vi "Sector Analysis Module.vi"(11 "Canceled?":bool) -> (2 "State":T1, 3 "Data":bool, 4 "Left Sector Edge":u8, 5 "Right Sector Edge":u8)   [LabVIEW 2013]
uses:
  Sector Analysis Module Enum.ctl
  <vilib>/rvi/FIFO/Fifo_Resource/nirvififoEmulationReadFpgaImpl.vi
  <vilib>/rvi/DataTransferAndStorage/Container/Common/niFpgaContainerGetUniqueNameForEmu.vi
  Globals/Sector Parameter Global.vi
  <vilib>/rvi/Emulation/niFpgaSctlEmulationGetInTimedLoop.vi
  <vilib>/rvi/Emulation/niFpgaProcessEmulError.vi
  Globals/Accumulated Sector Intensity.vi
  <vilib>/rvi/FIFO/Fifo_Resource/nirvififoEmulationClearFpgaImpl.vi
  <vilib>/rvi/DataTransferAndStorage/Container/XNode/niFpgaContainer.xnode
  <vilib>/rvi/FIFO/Fifo_Resource/nirvififoEmulationRead.vi
  <vilib>/rvi/FIFO/Fifo_Resource/nirvififoEmulationClear.vi
panel:
  out "2nd Analysis Left Sector":u8
  out "2nd Analysis Right Sector":u8
  out "Preanalysis Right Sector Edge":u8
  out "Preanalysis Left Sector Edge":u8
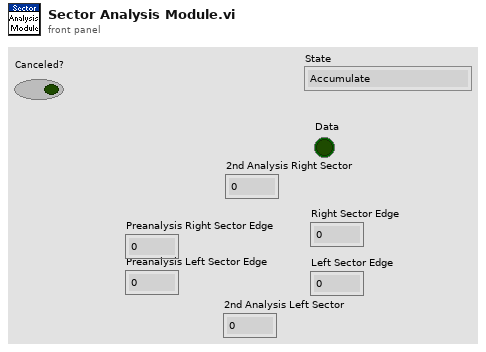
[diagram p1: front panel]
types:
  T1 = typedef "Sector Analysis Module Enum.ctl" = enum16{"Accumulate", "Analysis", "Reset"}
  T2 = typedef "Sector Parameter Cluster.ctl" = cluster{"Start Angle":fxp<+/-,17,2>, "End Angle":fxp<+/-,17,2>, "Inner Radius":u16, "Outter Radius":u16, "Hinge X":u16, "Hinge Y":u16, "NumWingSectors":u8}
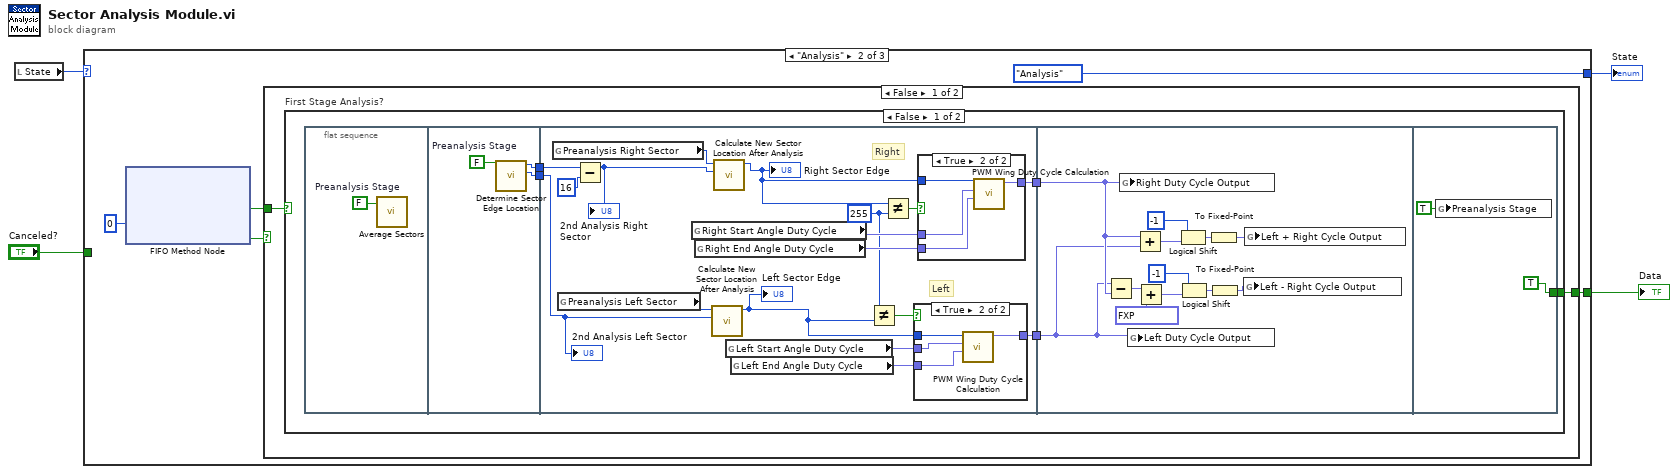
[diagram p0: block diagram]
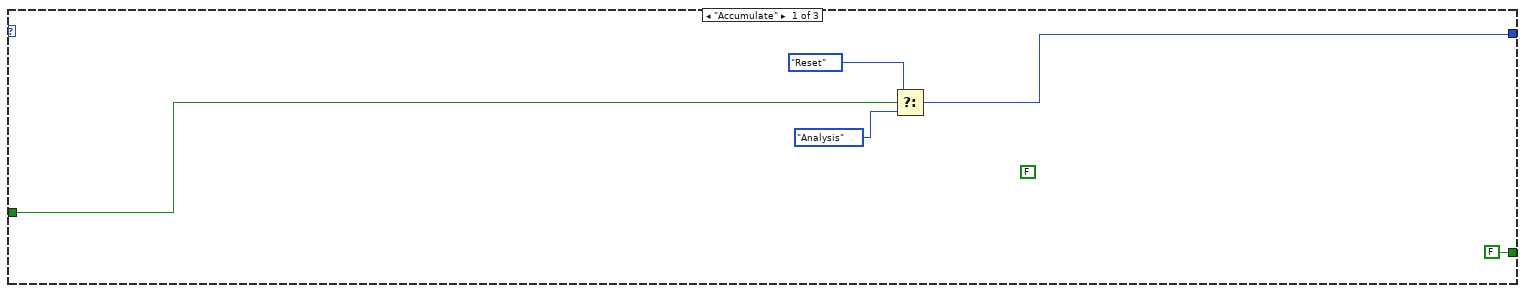
[diagram p2: hidden frame]
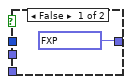
[diagram p3: hidden frame]
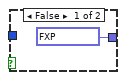
[diagram p4: hidden frame]
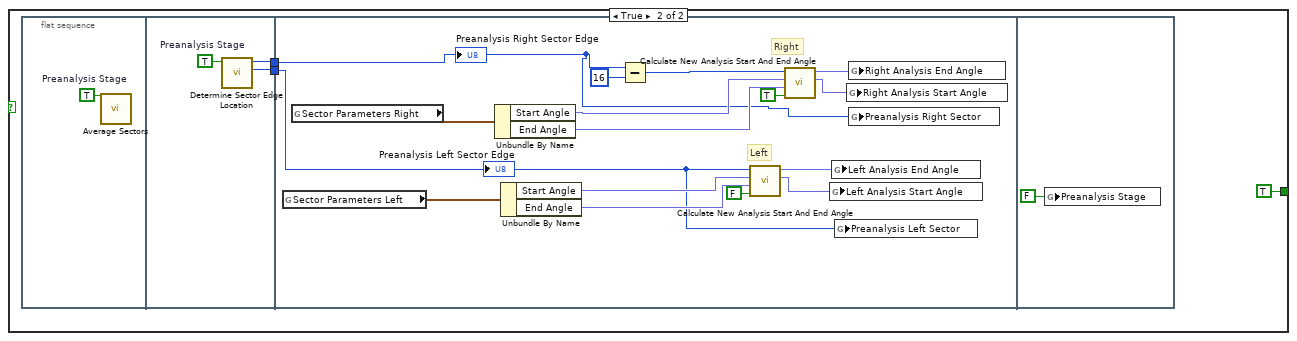
[diagram p5: hidden frame]
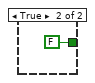
[diagram p6: hidden frame]
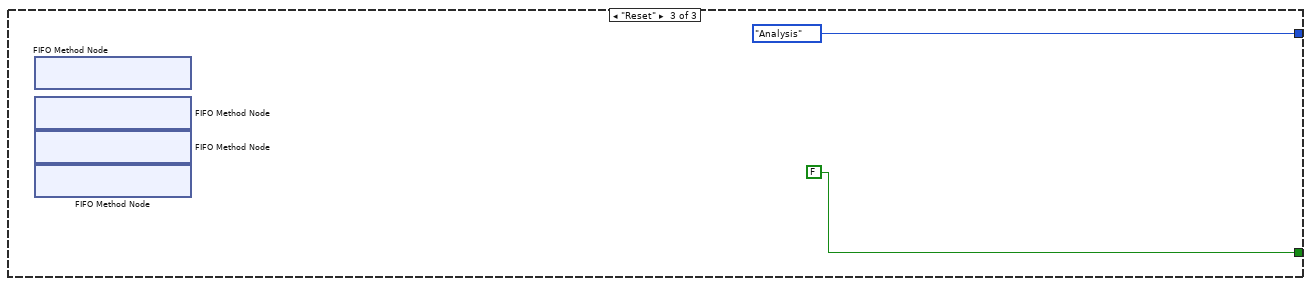
[diagram p7: hidden frame]
diagram:
  n1 = local read "State"() -> (w4:T1)
  n2 = case shown="\"Analysis\"" w4 {
    tunnel: [w8 Sector_Analysis_Module_Enum."Analysis" ("State") Sector_Analysis_Module_Enum."Analysis" ("State")] -> w3
    tunnel: "Canceled?" -> [w9 _ _]
    tunnel: [FALSE ("New Data? Out") w10 FALSE ("New Data? Out")] -> w1
    frame "Accumulate" {
      (unwired) FALSE ("New Data? Out")
      n3 = Select(t=Sector_Analysis_Module_Enum."Reset", s=w9, f=Sector_Analysis_Module_Enum."Analysis" ("State")) -> (s? t:f=w8:T1)
    }
    frame "Analysis" {
      n4 = xnode ("FIFO Method Node")("Timeout"=0) -> ("Element"=w11:bool, "Timed Out?"=w13:bool)  [unwired: 1 in, 1 out]
      n5 = case shown="False" w13 {
        tunnel: w11 -> [w16 _]
        tunnel: [w15 FALSE ("Data")] -> w10
        frame False {
          n6 = case "First Stage Analysis?" shown="False" w16 {
            tunnel: [w17 TRUE ("Data")] -> w15
            frame False {
              n7 = flat-sequence {
                tunnel: [w25] -> w20
                tunnel: [w24] -> w21
                tunnel: w21 -> [w29]
                tunnel: w20 -> [w32]
                tunnel: [w36] -> w19
                tunnel: [w35] -> w18
                tunnel: w19 -> [w54]
                tunnel: w18 -> [w55]
                tunnel: [TRUE ("Data")] -> w17
                frame #0 {
                  w22 = FALSE  # Preanalysis Stage
                  n8 = call "Average Sectors.vi"("Preanalysis Stage"=w22) -> ()  [unwired: 11 in]
                }
                frame #1 {
                  w23 = FALSE  # Preanalysis Stage
                  n9 = call "Determine Sector Edge Location.vi"("Preanalysis Stage"=w23) -> ("Left Sector Edge"=w24:u8, "Right Sector Edge"=w25:u8)  [unwired: 9 in]
                }
                frame #2 {
                  w33 = u8 255 ("y")
                  # "Left"
                  # "Right"
                  n10 = global read "Sector Parameter Global.vi" "Preanalysis Right Sector"() -> (w31:u8)
                  n11 = global read "Sector Parameter Global.vi" "Preanalysis Left Sector"() -> (w30:u8)
                  n12 = Subtract(x=w32, y=u8 16) -> (x-y=w28:u8)
                  "2nd Analysis Right Sector" <- w28
                  n13 = global read "Sector Parameter Global.vi" "Right Start Angle Duty Cycle"() -> (w41:fxp<+,8,0>)
                  n14 = global read "Sector Parameter Global.vi" "Right End Angle Duty Cycle"() -> (w40:fxp<+,8,0>)
                  n15 = call "Calculate New Sector Location After Analysis.vi"("2nd Analysis Sector"=w29, "Preanalysis Sector"=w30) -> ("New Sector"=w26:u8)  [unwired: 9 in]
                  "Left Sector Edge" <- w26
                  n16 = call "Calculate New Sector Location After Analysis.vi"("2nd Analysis Sector"=w28, "Preanalysis Sector"=w31) -> ("New Sector"=w34:u8)  [unwired: 9 in]
                  "Right Sector Edge" <- w34
                  n17 = global read "Sector Parameter Global.vi" "Left Start Angle Duty Cycle"() -> (w38:fxp<+,8,0>)
                  n18 = global read "Sector Parameter Global.vi" "Left End Angle Duty Cycle"() -> (w37:fxp<+,8,0>)
                  n19 = Not Equal?(x=w33, y=w26) -> (x != y?=w39:bool)
                  n20 = Not Equal?(x=w34, y=w33) -> (x != y?=w42:bool)
                  n21 = case shown="True" w39 {
                    tunnel: w26 -> [_ w47]
                    tunnel: w38 -> [_ w46]
                    tunnel: w37 -> [_ w45]
                    tunnel: [fxp<+,8,0> 0.99609375 ("Duty Cycle Out") w44] -> w36
                    frame False {
                    }
                    frame True {
                      n22 = call "PWM Wing Duty Cycle Calculation.vi"("End Angle Duty Cycle"=w45, "Start Angle Duty Cycle"=w46, "Sector"=w47) -> ("Duty Cycle Out"=w44:fxp<+/-,9,1>)  [unwired: 8 in]
                    }
                  }
                  n23 = case shown="True" w42 {
                    tunnel: w34 -> [_ w52]
                    tunnel: w41 -> [_ w51]
                    tunnel: w40 -> [_ w50]
                    tunnel: [fxp<+,8,0> 0.99609375 ("Duty Cycle Out") w49] -> w35
                    frame False {
                    }
                    frame True {
                      n24 = call "PWM Wing Duty Cycle Calculation.vi"("End Angle Duty Cycle"=w50, "Start Angle Duty Cycle"=w51, "Sector"=w52) -> ("Duty Cycle Out"=w49:fxp<+/-,9,1>)  [unwired: 8 in]
                    }
                  }
                  "2nd Analysis Left Sector" <- w29
                }
                frame #3 {
                  n25 = Subtract(x=w54, y=w55) -> (x-y=w62:fxp<+/-,10,2>)
                  n26 = global write "Sector Parameter Global.vi" "Right Duty Cycle Output"(w55) -> ()
                  n27 = global write "Sector Parameter Global.vi" "Left Duty Cycle Output"(w54) -> ()
                  n28 = Add(x=w55, y=w54) -> (x+y=w56:fxp<+/-,10,2>)
                  n29 = Add(x=w62, y=fxp<+/-,9,1> 0.99609375) -> (x+y=w64:fxp<+/-,11,3>)
                  n30 = Logical Shift(y=i16 -1, x=w56) -> (x << y=w58:fxp<+/-,10,2>)
                  n31 = Logical Shift(y=i16 -1, x=w64) -> (x << y=w60:fxp<+/-,11,3>)
                  n32 = To Fixed-Point(number=w58) -> (fixed-point=w53:fxp<+,8,0>)  [unwired: 1 in]
                  n33 = To Fixed-Point(number=w60) -> (fixed-point=w59:fxp<+,8,0>)  [unwired: 1 in]
                  n34 = global write "Sector Parameter Global.vi" "Left - Right Cycle Output"(w59) -> ()
                  n35 = global write "Sector Parameter Global.vi" "Left + Right Cycle Output"(w53) -> ()
                }
                frame #4 {
                  n36 = global write "Accumulated Sector Intensity.vi" "Preanalysis Stage"(TRUE ("Preanalysis Stage")) -> ()
                }
              }
            }
            frame True {
              n37 = flat-sequence {
                tunnel: [w73] -> w68
                tunnel: [w72] -> w69
                tunnel: w68 -> [w74]
                tunnel: w69 -> [w75]
                frame #0 {
                  w70 = TRUE  # Preanalysis Stage
                  n38 = call "Average Sectors.vi"("Preanalysis Stage"=w70) -> ()  [unwired: 11 in]
                }
                frame #1 {
                  w71 = TRUE  # Preanalysis Stage
                  n39 = call "Determine Sector Edge Location.vi"("Preanalysis Stage"=w71) -> ("Left Sector Edge"=w72:u8, "Right Sector Edge"=w73:u8)  [unwired: 9 in]
                }
                frame #2 {
                  # "Left"
                  # "Right"
                  n40 = global read "Sector Parameter Global.vi" "Sector Parameters Left"() -> (w83:T2)
                  n41 = global read "Sector Parameter Global.vi" "Sector Parameters Right"() -> (w87:T2)
                  n42 = Unbundle By Name(w87) -> ("Start Angle"=w86:fxp<+/-,17,2>, "End Angle"=w85:fxp<+/-,17,2>)
                  n43 = Unbundle By Name(w83) -> ("Start Angle"=w82:fxp<+/-,17,2>, "End Angle"=w81:fxp<+/-,17,2>)
                  n44 = Subtract(x=w74, y=u8 16) -> (x-y=w89:u8)
                  n45 = call "Calculate New Analysis Start And End Angle.vi"("Right Wing?"=FALSE, "End Angle"=w81, "Start Angle"=w82, "Sector"=w75) -> ("Start Angle Out"=w78:fxp<+/-,17,2>, "End Angle Out"=w79:fxp<+/-,17,2>)  [unwired: 6 in]
                  n46 = call "Calculate New Analysis Start And End Angle.vi"("Right Wing?"=TRUE, "End Angle"=w85, "Start Angle"=w86, "Sector"=w89) -> ("Start Angle Out"=w76:fxp<+/-,17,2>, "End Angle Out"=w77:fxp<+/-,17,2>)  [unwired: 6 in]
                  n47 = global write "Sector Parameter Global.vi" "Left Analysis Start Angle"(w78) -> ()
                  n48 = global write "Sector Parameter Global.vi" "Left Analysis End Angle"(w79) -> ()
                  n49 = global write "Sector Parameter Global.vi" "Preanalysis Left Sector"(w75) -> ()
                  n50 = global write "Sector Parameter Global.vi" "Right Analysis Start Angle"(w76) -> ()
                  n51 = global write "Sector Parameter Global.vi" "Right Analysis End Angle"(w77) -> ()
                  n52 = global write "Sector Parameter Global.vi" "Preanalysis Right Sector"(w74) -> ()
                  "Preanalysis Right Sector Edge" <- w74
                  "Preanalysis Left Sector Edge" <- w75
                }
                frame #3 {
                  n53 = global write "Accumulated Sector Intensity.vi" "Preanalysis Stage"(FALSE ("Preanalysis Stage")) -> ()
                }
              }
            }
          }
        }
        frame True {
        }
      }
    }
    frame "Reset" {
      n54 = xnode ("FIFO Method Node")() -> ()  [unwired: 1 in, 1 out]
      n55 = xnode ("FIFO Method Node")() -> ()  [unwired: 1 in, 1 out]
      n56 = xnode ("FIFO Method Node")() -> ()  [unwired: 1 in, 1 out]
      n57 = xnode ("FIFO Method Node")() -> ()  [unwired: 1 in, 1 out]
    }
  }
  "State" <- w3
  "Data" <- w1
